vi "DeleteMenu.vi"(8 "error in (no error)":errorcluster caption="错误输入（无错误）", 11 "listbox 输入":refnum<class "listbox.lvclass">) -> (0 "error out":errorcluster caption="错误输出", 3 "listbox 输出":refnum<class "listbox.lvclass">)   [LabVIEW 2016, in "listbox.lvclass"]
uses:
  listbox.lvclass
  listbox.lvclass/listbox.ctl
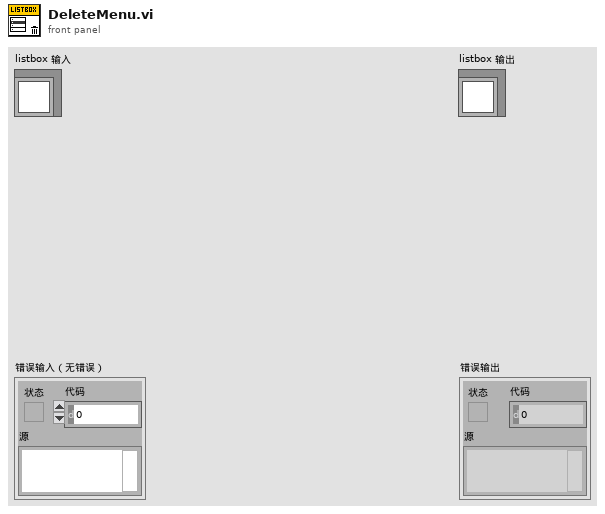
[diagram p1: front panel]
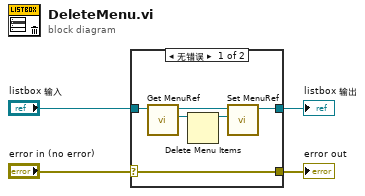
[diagram p0: block diagram]
diagram:
  n1 = case shown="无错误" "error in (no error)" {
    selector: "error in (no error)" -> [w9 w12]
    tunnel: [w9 w12] -> w3
    tunnel: [w7 w11] -> w1
    tunnel: "listbox 输入" -> [w10 w11]
    frame No Error {
      n2 = call "Get MenuRef.vi"("listbox in"=w10) -> ("MenuRef"=w6:refnum<k9>, "listbox out"=w8:refnum<class "listbox.lvclass">)  [unwired: 9 in]
      n3 = Delete Menu Items(9:w6) -> (3:w5:refnum<k9>)  [unwired: 3 in, 1 out]
      n4 = call "Set MenuRef.vi"("MenuRef"=w5, "listbox in"=w8) -> ("listbox out"=w7:refnum<class "listbox.lvclass">)  [unwired: 9 in]
    }
    frame Error {
    }
  }
  "error out" <- w3
  "listbox 输出" <- w1
